vi "8 (SubVI).vi"(11 "Scalar":dbl) -> (3 "Cluster":cluster{dbl[], dbl[]})   [LabVIEW 2020]
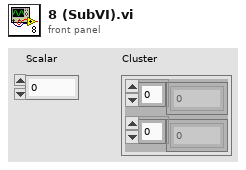
[diagram p1: front panel]
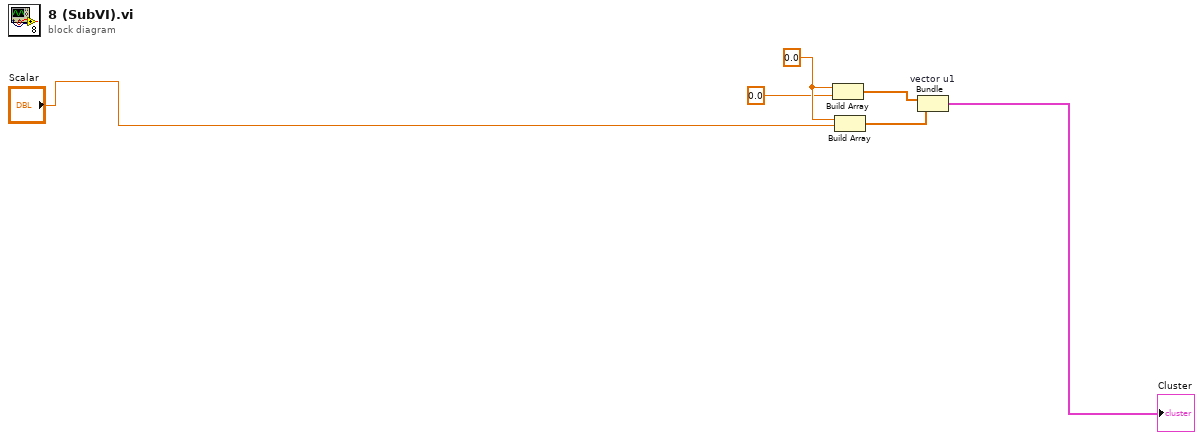
[diagram p0: block diagram]
diagram:
  w2 = 0.0 ("element")
  n1 = Build Array(w2, 0.0 ("element")) -> (w3:dbl[])
  n2 = Build Array(w2, "Scalar") -> (w4:dbl[])
  n3 = Bundle "vector u1"(w3, w4) -> (→"Cluster":cluster{dbl[], dbl[]})  [unwired: 1 in]
